vi "SetBaseClasses_DEPRECATED.vi"(0 "LibReader in":refnum<class "LibReader.lvclass">, 1 "Inheritance":path[](array[path]), 5 "error in (no error)":errorcluster) -> (14 "LibReader out":refnum<class "LibReader.lvclass">, 19 "error out":errorcluster)   [LabVIEW 2014]
uses:
  <resource>/Framework/Providers/Open_GDS/ClassProviders/LibProvider_BaseClassInterface/LibReader_class/LibReader.lvclass
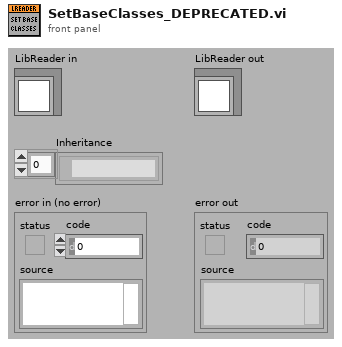
[diagram p1: front panel]
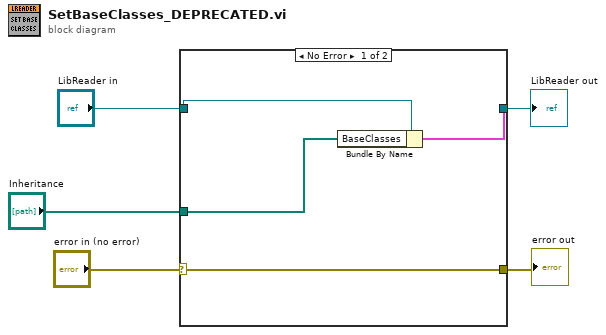
[diagram p0: block diagram]
diagram:
  n1 = case shown="No Error" "error in (no error)" {
    selector: "error in (no error)" -> [w6 w11]
    tunnel: [w6 w11] -> w4
    tunnel: [w8 w10] -> w2
    tunnel: "LibReader in" -> [w9 w10]
    tunnel: "Inheritance" -> [w7 _]
    frame No Error {
      n2 = Bundle By Name(cluster=w9, "BaseClasses"=w7) -> (w8:cluster{})
    }
    frame Error {
    }
  }
  "error out" <- w4
  "LibReader out" <- w2
